vi "solar_excel File Read (Sheet).vi"(4 "Truncate Empty Cells? (F)":bool, 6 "Visible? (F)":bool, 7 "Worksheet":string, 8 "error in (no error)":errorcluster, 9 "End (0,0 = Remaining)":cluster{"Row":u32, "Column":u32}, 10 "Start (1,1 = 'A1')":cluster{"Row":u32, "Column":u32}, 11 "Excel Workbook (*.xlsx)":path) -> (0 "error out":errorcluster, 2 "Cells":string[][](array[string]), 3 "dup Excel Workbook":path)   [LabVIEW 2018]
doc: "This returns cells from the specified Excel Workbook (*.xlsx) by <b>Start</b> and <b>End</b> cell ranges."
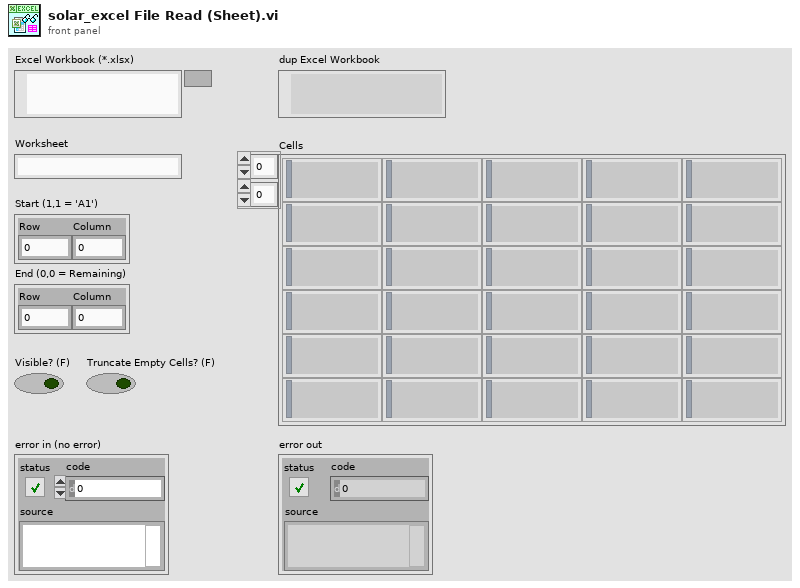
[diagram p1: front panel]
types:
  T1 = typedef "solar_excel_ctl App.ctl" = cluster{"ExcelApp":refnum<k7>, "Workbooks":refnum<k7>, "TSV":refnum<queue>}
  T2 = typedef "solar_excel_ctl Workbook.ctl" = cluster{"ExcelApp":refnum<k7>, "Workbooks":refnum<k7>, "TSV":refnum<queue>, "OpenWkb":refnum<k7>}
  T3 = typedef "solar_excel_ctl Worksheet.ctl" = cluster{"ExcelApp":refnum<k7>, "Workbooks":refnum<k7>, "TSV":refnum<queue>, "OpenWkb":refnum<k7>, "Worksheets":refnum<k7>, "OpenWksh":refnum<k7>}
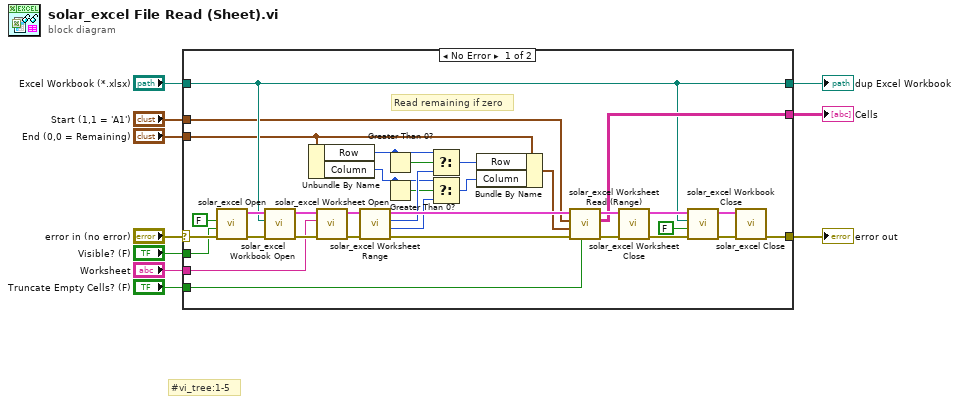
[diagram p0: block diagram]
diagram:
  # "#vi_tree:1-5"
  n1 = case shown="No Error" "error in (no error)" {
    selector: "error in (no error)" -> [w37 w46]
    tunnel: [w38 w46] -> w10
    tunnel: "Visible? (F)" -> [w36 _]
    tunnel: "Excel Workbook (*.xlsx)" -> [w22 w45]
    tunnel: [w24 _] -> w6
    tunnel: "Worksheet" -> [w23 _]
    tunnel: [w22 w45] -> w4
    tunnel: "Truncate Empty Cells? (F)" -> [w21 _]
    tunnel: "Start (1,1 = 'A1')" -> [w20 _]
    tunnel: "End (0,0 = Remaining)" -> [w19 _]
    frame No Error {
      # "Read remaining if zero"
      n2 = call "solar_excel Open.vi"("error in (no error)"=w37, "Visible? (F)"=w36, "Open New Instance? (F)"=FALSE) -> ("error out"=w43:errorcluster, "Excel App"=w44:T1)  [unwired: 7 in]
      n3 = call "solar_excel Workbook Open.vi"("error in (no error)"=w43, "Excel Workbook (*.xlsx)"=w22, "Excel App"=w44) -> ("error out"=w32:errorcluster, "Excel Workbook"=w33:T2)  [unwired: 7 in]
      n4 = Unbundle By Name(w19) -> ("Row"=w17:u32, "Column"=w13:u32)
      n5 = call "solar_excel Worksheet Open.vi"("error in (no error)"=w32, "Sheet Name (STR) or Number (I32)"=w23, "Excel Workbook"=w33) -> ("error out"=w31:errorcluster, "Excel Worksheet"=w30:T3)  [unwired: 5 in, 2 out]
      n6 = call "solar_excel Worksheet Range.vi"("error in (no error)"=w31, "Excel Worksheet in"=w30) -> ("error out"=w29:errorcluster, "Columns"=w12:u32, "Rows"=w16:u32, "Excel Worksheet out"=w28:T3)  [unwired: 6 in]
      n7 = Greater Than 0?(x=w17) -> (x > 0?=w18:bool)
      n8 = Greater Than 0?(x=w13) -> (x > 0?=w14:bool)
      n9 = Select(t=w17, s=w18, f=w16) -> (s? t:f=w15:u32)
      n10 = Select(t=w13, s=w14, f=w12) -> (s? t:f=w11:u32)
      n11 = Bundle By Name(cluster=w19, "Row"=w15, "Column"=w11) -> (w25:cluster{"Row":u32, "Column":u32})
      n12 = call "solar_excel Worksheet Read (Range).vi"("Truncate Empty Cells? (F)"=w21, "error in (no error)"=w29, "End (1,1 = 'A1')"=w25, "Start (1,1 = 'A1')"=w20, "Excel Worksheet in"=w28) -> ("error out"=w27:errorcluster, "Cells"=w24:string[][], "Excel Worksheet out"=w26:T3)  [unwired: 4 in]
      n13 = call "solar_excel Worksheet Close.vi"("error in (no error)"=w27, "Excel Worksheet"=w26) -> ("error out"=w42:errorcluster, "Excel Workbook"=w41:T2)  [unwired: 8 in]
      n14 = call "solar_excel Workbook Close.vi"("error in (no error)"=w42, "Save? (F)"=FALSE, "Excel Workbook (*.xlsx)"=w22, "Excel Workbook"=w41) -> ("error out"=w40:errorcluster, "Excel App"=w39:T1)  [unwired: 6 in]
      n15 = call "solar_excel Close.vi"("error in (no error)"=w40, "Excel App"=w39) -> ("error out"=w38:errorcluster)  [unwired: 9 in]
    }
    frame Error {
    }
  }
  "error out" <- w10
  "dup Excel Workbook" <- w4
  "Cells" <- w6
